vi "Actor Core.vi"(8 "error in":errorcluster, 11 "Timed Loop Controller":refnum<class "Timed Loop Actor.lvclass">) -> (0 "error out":errorcluster, 3 "Actor out":refnum<class "Actor.lvclass">)   [LabVIEW 2018, in "Timed Loop Actor.lvlib" / "Timed Loop Actor.lvclass"]
doc: "This is Actor Core.vi, the main message handling loop for Actors. An actor usually just sits in this loop and processes messages as they arrive. Any error returned by the message Do.vi call will stop the loop, with error code 43 as the canonical signal to stop with no error sent to caller. Descendants may override that in Handle Error.vi."
uses:
  Timed Loop Actor.lvclass
  C:/Program Files (x86)/National Instruments/LabVIEW 2018/vi.lib/ActorFramework/Actor/Actor.lvclass
  <vilib>/ActorFramework/Actor/Actor.lvclass
  <vilib>/ActorFramework/Actor/Actor.lvclass/Actor.ctl
  <vilib>/ActorFramework/Message Enqueuer/Message Enqueuer.lvclass/Message Enqueuer.ctl
  Timed Loop Actor.lvclass/Timed Loop Actor.ctl
  <vilib>/ActorFramework/Message Enqueuer/Init from Existing Queue.vi
  <vilib>/ActorFramework/Message Enqueuer/Enqueue.vi
  Update Msg/Update Msg.lvclass
  C:/Program Files (x86)/National Instruments/LabVIEW 2018/vi.lib/ActorFramework/Message/Message.lvclass
  <vilib>/Utility/LVClass/Get LV Class Path.vi
  <vilib>/ActorFramework/Message Priority Queue/Priority Enqueue.vi
  <vilib>/ActorFramework/Message Enqueuer/Message Enqueuer.lvclass
  <vilib>/Platform/TimedLoop/XDataNode/XDataNode.xnode
  <vilib>/Platform/TimedLoop/XDataNode/timing_clust.ctl
  <vilib>/Platform/TimedLoop/XDataNode/XDNodeRunTimeDep.lvlib
  <vilib>/Platform/TimedLoop/XDataNode/wakeup.ctl
  <vilib>/Platform/TimedLoop/XDataNode/nitl_modes.ctl
panel:
  in  "stop?":bool
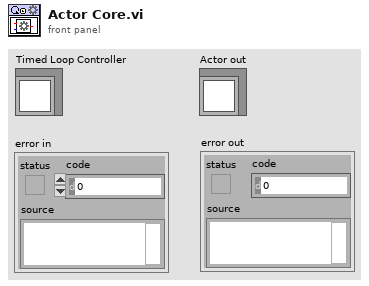
[diagram p1: front panel]
types:
  T1 = typedef "XDNodeRunTimeDep.lvlib/timing_clust.ctl" = cluster{"Expected End [f-1]":u64, "Actual End [f-1]":u64, "Finished Late? [f-1]":bool, "Expected End [i-1]":u64, "Actual End [i-1]":u64, "Finished Late? [i-1]":bool, "Expected Start [i]":u64, "Actual Start [i]":u64, "Expected Start [f]":u64, "Actual Start [f]":u64, "Source Name":string, "Structure Name":string, "Period":i64, "Deadline":i64, "Offset":i64, "Start":i64, "Priority":i32, "Timeout":i32, "Mode":T2, "Wakeup Reason":T3, "Error":errorcluster, "Source Type":string, "Secondary Source Type":string, "Global End Time":u64, "Global Start Time":u64, "Frame Duration":u64, "Iteration Duration":u64, "Assigned CPU":i32, "I/O Scan Engine Mode":u32}
  T2 = typedef "XDNodeRunTimeDep.lvlib/nitl_modes.ctl" = enum32{"No Change", "Process missed periods, maintain original phase", "Discard missed periods, maintain original phase", "Process missed periods, ignore original phase", "Discard missed periods, ignore original phase"}
  T3 = typedef "XDNodeRunTimeDep.lvlib/wakeup.ctl" = enum32{"Normal", "Aborted", "Asynchronous wakeup", "Timing source error", "Timed loop error", "Timeout"}
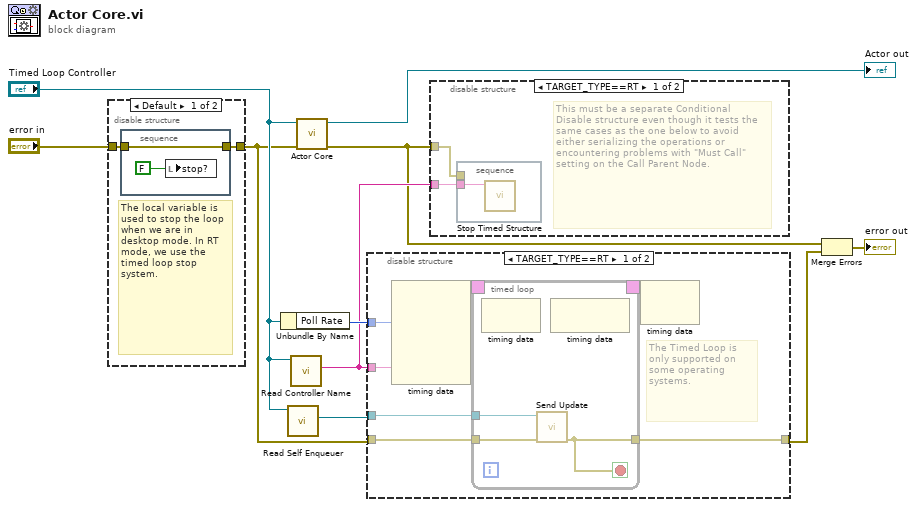
[diagram p0: block diagram]
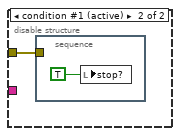
[diagram p3: hidden frame]
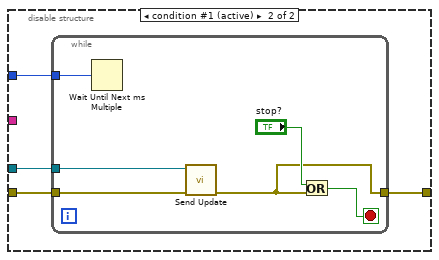
[diagram p4: hidden frame]
diagram:
  n1 = disable-structure shown="Default" {
    disable-tunnel: [w12 _] -> w2
    disable-tunnel: "error in" -> [w11 _]
    frame condition #0 (active) {
      # "The local variable is used to stop the loop when we are in desktop mode. In RT mode, we use the timed loop stop system."
      n2 = stacked-sequence {
        tunnel: [w13] -> w12
        tunnel: w11 -> [w13]
        frame #0 {
          n3 = local write "stop?"(FALSE) -> ()
        }
      }
    }
    frame condition #1 {
    }
  }
  n4 = Unbundle By Name("Timed Loop Controller") -> ("Poll Rate"=w9:i64)
  n5 = call <vilib>:"Read Self Enqueuer.vi"("Actor"="Timed Loop Controller") -> ("Self Enqueuer"=w10:refnum<class "Message Enqueuer.lvclass">)  [unwired: 10 in]
  n6 = call "Read Controller Name.vi"("Timed Loop Controller"="Timed Loop Controller") -> ("Controller Name"=w7:string)  [unwired: 10 in]
  n7 = call-parent "Actor Core.vi"("error in"=w2, "Actor in"="Timed Loop Controller") -> ("error out"=w5:errorcluster, "Actor out"=→"Actor out":refnum<class "Actor.lvclass">)  [unwired: 8 in]
  n8 = disable-structure shown="TARGET_TYPE==RT" {
    disable-tunnel: w10 -> [w19 w35]
    disable-tunnel: w9 -> [w18 w34]
    disable-tunnel: w7 -> [w17 _]
    disable-tunnel: w2 -> [w16 w33]
    disable-tunnel: [w15 w32] -> w4
    frame condition #0 {
      # "The Timed Loop is only supported on some operating systems."
      n9 = node-c288(w18, w17) -> (w21:T1)  [unwired: 3 in]
      n10 = timed-loop {
        timing: w21 -> [_]
        timing-out: [_] -> w20
        tunnel: w19 -> [w24]
        tunnel: w16 -> [w23]
        tunnel: [w22] -> w15
        stop <- w22 stop-if-true
        n11 = node-c288() -> ()  [unwired: 1 in, 1 out]
        n12 = call "Send Update.vi"("error in (no error)"=w23, "Message Enqueuer"=w24) -> ("error out"=w22:errorcluster)  [unwired: 9 in]
        n13 = node-c288() -> ()  [unwired: 1 in, 1 out]
      }
      n14 = node-c288(w20) -> ()  [unwired: 1 out]
    }
    frame condition #1 (active) {
      n15 = while {
        tunnel: w35 -> [w41]
        tunnel: w34 -> [w40]
        tunnel: w33 -> [w39]
        tunnel: [w36] -> w32
        stop <- w37 stop-if-true
        n16 = Wait Until Next ms Multiple(millisecond multiple=w40) -> ()  [unwired: 1 out]
        n17 = call "Send Update.vi"("error in (no error)"=w39, "Message Enqueuer"=w41) -> ("error out"=w36:errorcluster)  [unwired: 9 in]
        n18 = Or(x="stop?", y=w36) -> (x .or. y?=w37:bool)
      }
    }
  }
  n19 = disable-structure shown="TARGET_TYPE==RT" {
    disable-tunnel: w5 -> [w42 w45]
    disable-tunnel: w7 -> [w43 _]
    frame condition #0 {
      # "This must be a separate Conditional Disable structure even though it tests the same cases as the one below to avoid either serializing the operations or encountering problems with \"Must Call\" setting on the Call Parent Node."
      n20 = stacked-sequence {
        tunnel: w43 -> [w44]
        tunnel: w42 -> [_]
        frame #0 {
          n21 = call <vilib>:"Stop Timed Structure.vi"("name"=w44) -> ()  [unwired: 10 in, 1 out]
        }
      }
    }
    frame condition #1 (active) {
      n22 = stacked-sequence {
        tunnel: w45 -> [_]
        frame #0 {
          n23 = local write "stop?"(TRUE) -> ()
        }
      }
    }
  }
  n24 = Merge Errors(w5, w4) -> (→"error out":errorcluster)
